vi "Initial Values-format and values-Ref window.vi"() -> (13 "Values.Boolean":bool[](array[boolean]), 14 "Keys setup.DBL":T2=[{"key"="Control FPGA.Clock Freq (MHz)", "Save?"=TRUE, "Default"=240.0}, {"key"="DAQ FPGA.Clock Freq (MHz)", "Save?"=TRUE, "Default"=240.0}], 15 "Values.DBL":dbl[](array[numeric]), 16 "Keys setup.String":T3=[{"key"="Control FPGA.MAC address", "Save?"=TRUE, "Default"="AABBCCDDEEFF"}, {"key"="DAQ FPGA.Target", "Save?"=TRUE, "Default"="RIO0"}, {"key"="XY Stage.COM port", "Save?"=TRUE, "Default"="COM7"}, {"key"="DAQmx Chan.Pockels Control", "Save?"=TRUE, "Default"=""}, {"key"="DAQmx Chan.Hard Shutter", "Save?"=TRUE, "Default"=""}, {"key"="DAQmx Chan.PMT 1", "Save?"=TRUE, "Default"=""}, {"key"="DAQmx Chan.PMT 2", "Save?"=TRUE, "Default"=""}, {"key"="DAQmx Chan.Encoder Trigger", "Save?"=TRUE, "Default"=""}, {"key"="DAQmx Chan.Optional Trigger 1", "Save?"=TRUE, "Default"=""}, {"key"="DAQmx Chan.Optional Trigger 2", "Save?"=TRUE, "Default"=""}, {"key"="DAQmx Chan.Optional Trigger 3", "Save?"=TRUE, "Default"=""}], 17 "Values.Strings":string[](array[string]), 18 "Keys setup.Boolean":T1, 19 "error out":errorcluster)   [LabVIEW 2020]
uses:
  Typedefs/Ini file interface (String).ctl
  Typedefs/Ini file interface (DBL).ctl
  Typedefs/Ini file interface (Boolean).ctl
  User Interface/Globals/gl_Windows Ctrl refs.vi
panel:
  # "NOTES:\n1. \"Control FPGA.Ethernet port\" is detected automatically. It is not saved/loaded from file.\n2. \"Control FPGA.Ethernet Opened\" is detected automatically. It is not saved/loaded from file."
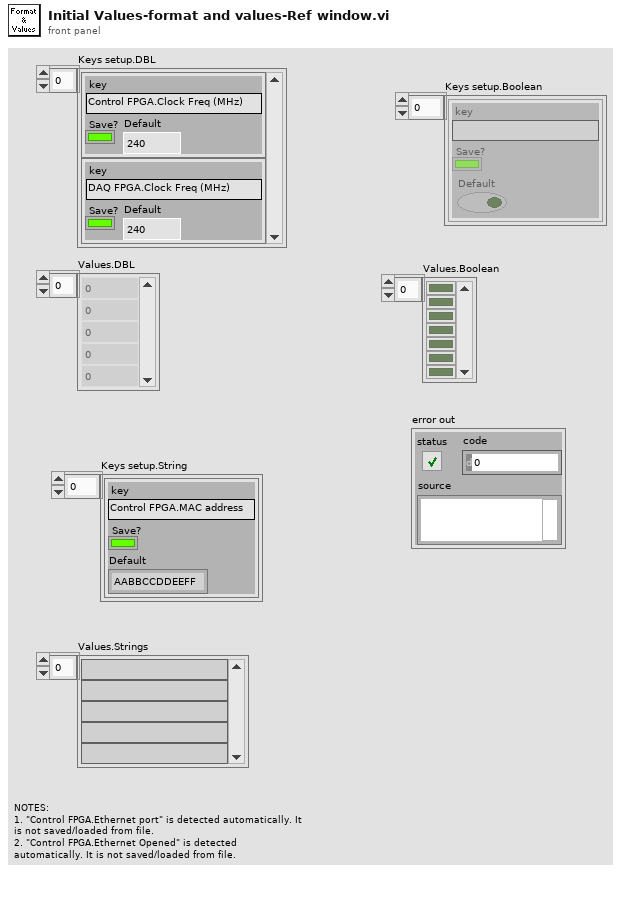
[diagram p1: front panel]
types:
  T1 = typedef "Ini file interface (Boolean).ctl" = cluster{"key":string, "Save?":bool, "Default":bool}[]
  T2 = typedef "Ini file interface (DBL).ctl" = cluster{"key":string, "Save?":bool, "Default":dbl}[]
  T3 = typedef "Ini file interface (String).ctl" = cluster{"key":string, "Save?":bool, "Default":string}[]
  T4 = typedef "Live window-ctrl refs.ctl" = cluster{"This VI":refnum<vi>, "Pane":refnum<vi>, "Show REF Image Left":refnum<vi>, "Show REF Image Right":refnum<vi>, "Snapshot":refnum<vi>, "Left Image Palette":refnum<vi>, "Right Image Palette":refnum<vi>, "Left Channel":refnum<vi>, "Right Channel":refnum<vi>, "Left image intensity":refnum<vi>, "Right image intensity":refnum<vi>, "Left Image Display":T5, "Right Image Display":T5, "Refresh rate ind (Hz)":refnum<vi>, "Acq rate ind (Hz)":refnum<vi>, "Stop (ind)":refnum<vi>}
  T5 = typedef "Image display ref.ctl" = refnum<vi>
  T6 = typedef "Channel Selector.ctl" = enum16{"Red Channel", "Green Channel", "Blended"}
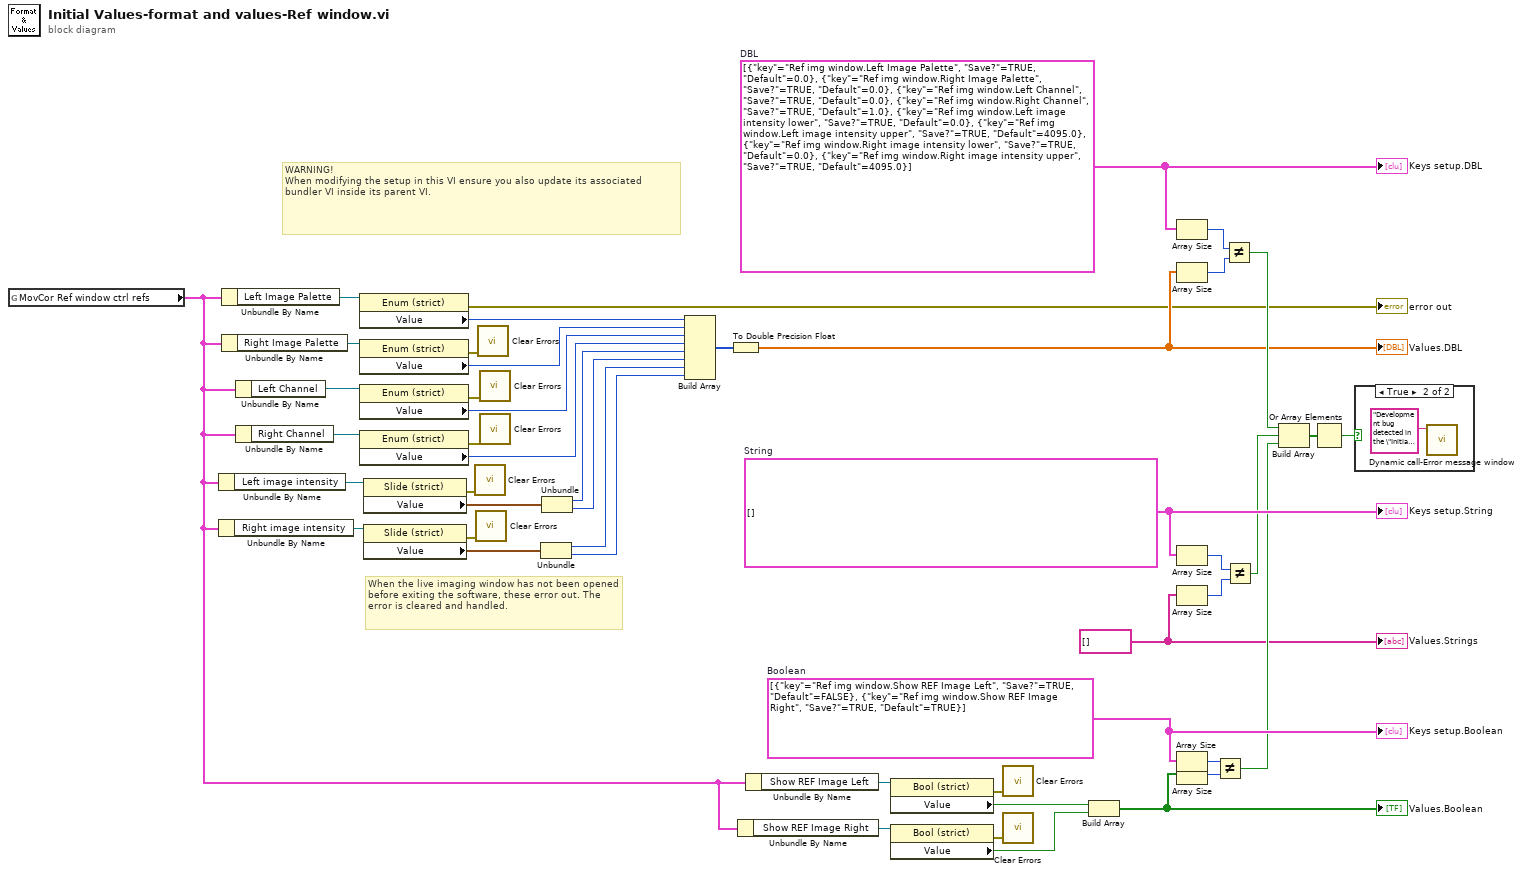
[diagram p0: block diagram]
diagram:
  w31 = string[] [] ("appended array")
  w44 = T1 [{"key"="Ref img window.Show REF Image Left", "Save?"=TRUE, "Default"=FALSE}, {"key"="Ref img window.Show REF Image Right", "Save?"=TRUE, "Default"=TRUE}]  # Boolean
  w47 = T3 []  # String
  w46 = T2 [{"key"="Ref img window.Left Image Palette", "Save?"=TRUE, "Default"=0.0}, {"key"="Ref img window.Right Image Palette", "Save?"=TRUE, "Default"=0.0}, {"key"="Ref img window.Left Channel", "Save?"=TRUE, "Default"=0.0}, {"key"="Ref img window.Right Channel", "Save?"=TRUE, "Default"=1.0}, {"key"="Ref img window.Left image intensity lower", "Save?"=TRUE, "Default"=0.0}, {"key"="Ref img window.Left image intensity upper", "Save?"=TRUE, "Default"=4095.0}, {"key"="Ref img window.Right image intensity lower", "Save?"=TRUE, "Default"=0.0}, {"key"="Ref img window.Right image intensity upper", "Save?"=TRUE, "Default"=4095.0}]  # DBL
  # "When the live imaging window has not been opened before exiting the software, these error out. The error is cleared and handled."
  # "WARNING!\nWhen modifying the setup in this VI ensure you also update its associated bundler VI inside its parent VI."
  n1 = global read "gl_Windows Ctrl refs.vi" "MovCor Ref window ctrl refs"() -> (w1:T4)
  n2 = Unbundle By Name(w1) -> ("Left image intensity"=w21:refnum<vi>)
  n3 = Unbundle By Name(w1) -> ("Right image intensity"=w22:refnum<vi>)
  n4 = Unbundle By Name(w1) -> ("Left Image Palette"=w32:refnum<vi>)
  n5 = Unbundle By Name(w1) -> ("Right Image Palette"=w29:refnum<vi>)
  n6 = Unbundle By Name(w1) -> ("Left Channel"=w26:refnum<vi>)
  n7 = Unbundle By Name(w1) -> ("Right Channel"=w27:refnum<vi>)
  n8 = property class="Enum (strict)"(reference=w32) -> (error out=→"error out":errorcluster, "Value"=w30:enum16{"Gray", "Red", "Green"})  [unwired: 1 in, 1 out]
  n9 = property class="Enum (strict)"(reference=w29) -> (error out=w14:errorcluster, "Value"=w28:enum16{"Gray", "Red", "Green"})  [unwired: 1 in, 1 out]
  n10 = property class="Enum (strict)"(reference=w26) -> (error out=w13:errorcluster, "Value"=w25:T6)  [unwired: 1 in, 1 out]
  n11 = property class="Enum (strict)"(reference=w27) -> (error out=w12:errorcluster, "Value"=w24:T6)  [unwired: 1 in, 1 out]
  n12 = property class="Slide (strict)"(reference=w21) -> (error out=w11:errorcluster, "Value"=w20:cluster{i16, i16})  [unwired: 1 in, 1 out]
  n13 = property class="Slide (strict)"(reference=w22) -> (error out=w10:errorcluster, "Value"=w19:cluster{i16, i16})  [unwired: 1 in, 1 out]
  n14 = call <vilib>:"Clear Errors.vi"("error in (no error)"=w11) -> ()  [unwired: 5 in, 2 out]
  n15 = call <vilib>:"Clear Errors.vi"("error in (no error)"=w10) -> ()  [unwired: 5 in, 2 out]
  n16 = call <vilib>:"Clear Errors.vi"("error in (no error)"=w14) -> ()  [unwired: 5 in, 2 out]
  n17 = call <vilib>:"Clear Errors.vi"("error in (no error)"=w13) -> ()  [unwired: 5 in, 2 out]
  n18 = call <vilib>:"Clear Errors.vi"("error in (no error)"=w12) -> ()  [unwired: 5 in, 2 out]
  n19 = Unbundle(w19) -> (w16:i16, w15:i16)
  n20 = Unbundle(w20) -> (w18:i16, w17:i16)
  n21 = Build Array(w30, w28, w25, w24, w18, w17, w16, w15) -> (w45:u16[])
  n22 = To Double Precision Float(number=w45) -> (double precision float=w23:dbl[])
  "Values.DBL" <- w23
  n23 = Unbundle By Name(w1) -> ("Show REF Image Right"=w8:refnum<vi>)
  n24 = Unbundle By Name(w1) -> ("Show REF Image Left"=w7:refnum<vi>)
  n25 = property class="Bool (strict)"(reference=w7) -> (error out=w3:errorcluster, "Value"=w6:bool)  [unwired: 1 in, 1 out]
  n26 = property class="Bool (strict)"(reference=w8) -> (error out=w2:errorcluster, "Value"=w5:bool)  [unwired: 1 in, 1 out]
  n27 = call <vilib>:"Clear Errors.vi"("error in (no error)"=w3) -> ()  [unwired: 5 in, 2 out]
  n28 = call <vilib>:"Clear Errors.vi"("error in (no error)"=w2) -> ()  [unwired: 5 in, 2 out]
  n29 = Build Array(w6, w5) -> (w4:bool[])
  "Values.Boolean" <- w4
  n30 = Array Size(array=w46) -> (size(s)=w41:i32)
  n31 = Array Size(array=w23) -> (size(s)=w40:i32)
  n32 = Array Size(array=w47) -> (size(s)=w43:i32)
  n33 = Array Size(array=w31) -> (size(s)=w42:i32)
  n34 = Array Size(array=w44) -> (size(s)=w39:i32)
  n35 = Array Size(array=w4) -> (size(s)=w38:i32)
  n36 = Not Equal?(x=w39, y=w38) -> (x != y?=w36:bool)
  n37 = Not Equal?(x=w41, y=w40) -> (x != y?=w34:bool)
  n38 = Not Equal?(x=w43, y=w42) -> (x != y?=w33:bool)
  n39 = Build Array(w34, w33, w36) -> (w37:bool[])
  n40 = Or Array Elements(Boolean array=w37) -> (logical OR=w35:bool)
  n41 = case shown="True" w35 {
    frame False {
    }
    frame True {
      n42 = call "Dynamic call-Error message window.vi"("Error Message"="Development bug detected in the \"Initial Values-format and values-Ref window.vi\".\nPlease correct the set up in this VI.") -> ()  [unwired: 10 in, 1 out]
    }
  }
  "Keys setup.String" <- w47
  "Keys setup.DBL" <- w46
  "Values.Strings" <- w31
  "Keys setup.Boolean" <- w44
